vi "sq_root_case(1).vi"() -> ()   [LabVIEW 2014]
panel:
  out "Result":dbl
  in  "Number Selector":dbl
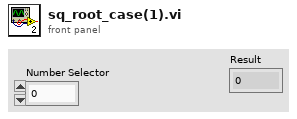
[diagram p1: front panel]
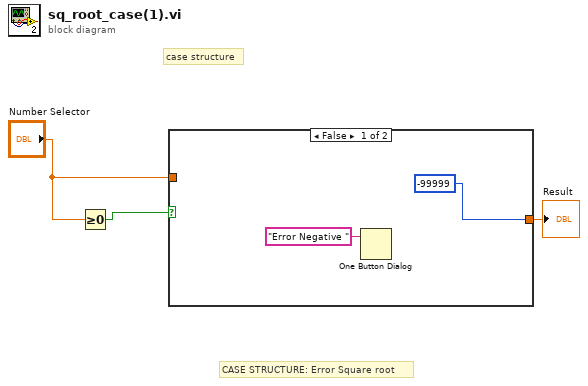
[diagram p0: block diagram]
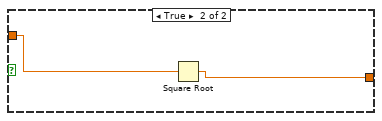
[diagram p2: hidden frame]
diagram:
  # "case structure"
  # "CASE STRUCTURE: Error Square root"
  n1 = Greater Or Equal To 0?(x="Number Selector") -> (x >= 0?=w3:bool)
  n2 = case shown="False" w3 {
    tunnel: "Number Selector" -> [_ w7]
    tunnel: [-99999 w6] -> w1
    frame False {
      n3 = One Button Dialog(message="Error Negative ") -> ()  [unwired: 1 in, 1 out]
    }
    frame True {
      n4 = Square Root(x=w7) -> (sqrt(x)=w6:dbl)
    }
  }
  "Result" <- w1
